vi "NI VeriStand - Initialize cRIO Timing Engine.vi"(9 "Use External Timing In":bool, 10 "Write to  RTSI In":bool) -> (1 "Use External Timing Out":bool, 2 "Write to  RTSI Out":bool)   [LabVIEW 2010, in "NI_VS FPGA Clock Support.lvlib"]
uses:
  <userlib>/_NI VeriStand FPGA Support/NI VeriStand FPGA Clock Support/NI_VS FPGA Clock Support.lvlib
  <userlib>/_NI VeriStand FPGA Support/NI VeriStand FPGA Clock Support/NI VeriStand - Timing Engine Globals.vi
  <vilib>/eio/EIONode/EIONode.xnode
  <vilib>/eio/EIOMethodNode/EIOMethodNode.xnode
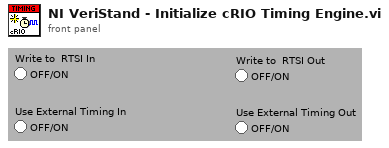
[diagram p1: front panel]
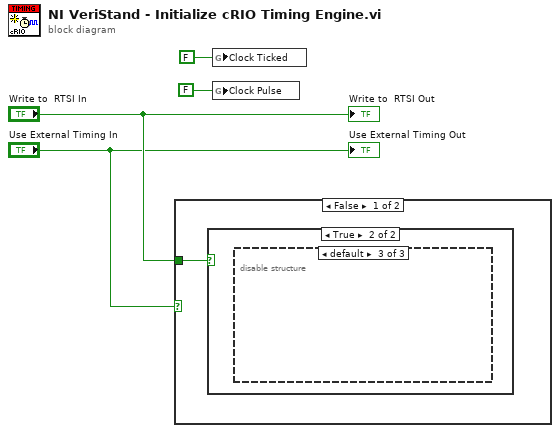
[diagram p0: block diagram]
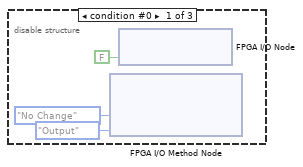
[diagram p3: hidden frame]
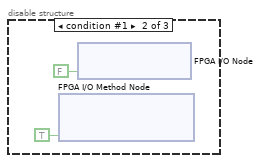
[diagram p4: hidden frame]
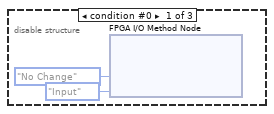
[diagram p6: hidden frame]
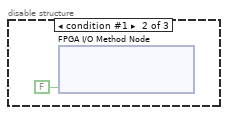
[diagram p7: hidden frame]
diagram:
  n1 = case shown="False" "Use External Timing In" {
    tunnel: "Write to  RTSI In" -> [w5 _]
    frame False {
      n2 = case shown="True" w5 {
        frame False {
        }
        frame True {
          n3 = disable-structure shown="default" {
            frame condition #0 {
              n4 = xnode "FPGA I/O Method Node"("DIO 7:4"=enum8{"No Change", "Input", "Output"}."No Change", "DIO 3:0"=enum8{"No Change", "Input", "Output"}."Output") -> ()  [unwired: 1 in, 1 out]
              n5 = xnode "FPGA I/O Node"("NI 9401/DIO0"=FALSE ("TRIG0")) -> ()  [unwired: 1 in, 1 out]
            }
            frame condition #1 {
              n6 = xnode "FPGA I/O Method Node"("Enable"=TRUE) -> ()  [unwired: 1 in, 1 out]
              n7 = xnode "FPGA I/O Node"("NI 9402/DIO0"=FALSE ("TRIG0")) -> ()  [unwired: 1 in, 1 out]
            }
            frame condition #2 (active) {
            }
          }
        }
      }
    }
    frame True {
      n8 = disable-structure shown="default" {
        frame condition #0 {
          n9 = xnode "FPGA I/O Method Node"("DIO 7:4"=enum8{"No Change", "Input", "Output"}."No Change", "DIO 3:0"=enum8{"No Change", "Input", "Output"}."Input") -> ()  [unwired: 1 in, 1 out]
        }
        frame condition #1 {
          n10 = xnode "FPGA I/O Method Node"("Enable"=FALSE) -> ()  [unwired: 1 in, 1 out]
        }
        frame condition #2 (active) {
        }
      }
    }
  }
  n11 = global write "NI VeriStand - Timing Engine Globals.vi" "Clock Ticked"(FALSE ("Clock Ticked")) -> ()
  n12 = global write "NI VeriStand - Timing Engine Globals.vi" "Clock Pulse"(FALSE ("Clock Ticked")) -> ()
  "Write to  RTSI Out" <- "Write to  RTSI In"
  "Use External Timing Out" <- "Use External Timing In"
